vi "Declare_Sync_Client.vi"   [LabVIEW 2020]
uses:
  ADAM Client/Sub VIs/ADAM Controls/Channel_State.ctl
  ADAM Client/Sub VIs/ADAM Controls/Calib_type_ADAM.ctl
  ADAM Client/Sub VIs/ADAM Controls/Module_type_ADAM.ctl
  ADAM Client/Sub VIs/ADAM Controls/Ch_description_ADAM.ctl
  ADAM Client/Sub VIs/ADAM Controls/Function_ADAM.ctl
  ADAM Client/Sub VIs/ADAM Controls/Address.ctl
  ADAM Client/Sub VIs/ADAM Controls/Update_scan_value.ctl
  Globals/Preference_global.vi
types:
  T1 = typedef "Channel_State.ctl" = enum16{"On", "Off", "Always On", "Always Off"}
  T2 = typedef "Ch_description_ADAM.ctl" = cluster{"Ch Name":string, "Type":T3, "Function":T4, "Ch State":T1, "Calibration type":T5, "A":dbl, "B":dbl, "C":dbl, "D":dbl, "Comments":string, "Address":T6, "String":string, "Duty":u16}
  T3 = typedef "Module_type_ADAM.ctl" = string
  T4 = typedef "Function_ADAM.ctl" = enum16{"Analogue Input", "Digital Input", "Event counter", "Event rate", "Analogue Output", "Digital Output", "Relay Output"}
  T5 = typedef "Calib_type_ADAM.ctl" = string
  T6 = typedef "Address.ctl" = cluster{"Main":i32, "Ch.":i32, "Sub":i32, "Port Name":string}
  T7 = typedef "Update_scan_value.ctl" = cluster{"Channel Name":string, "New Value":dbl}
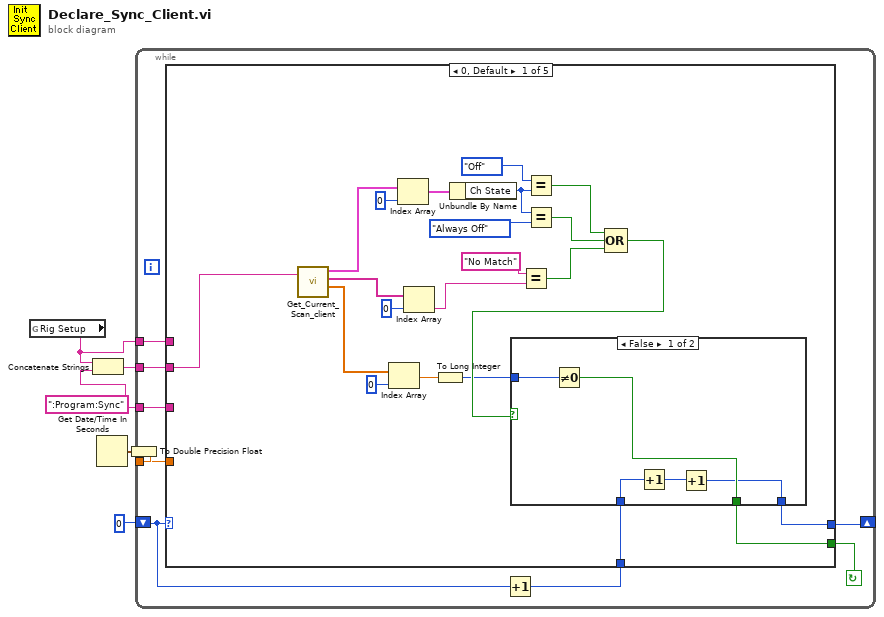
[diagram p0: block diagram]
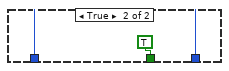
[diagram p2: hidden frame]
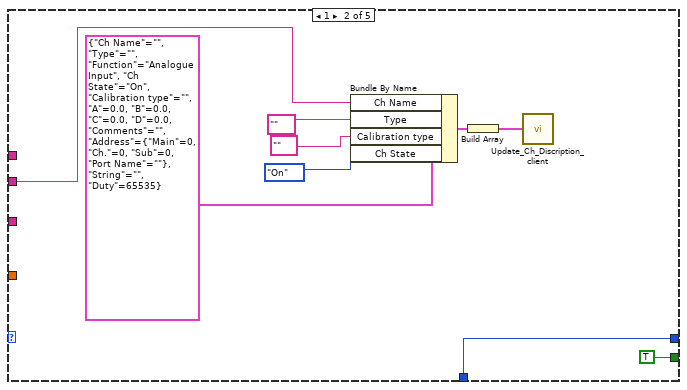
[diagram p3: hidden frame]
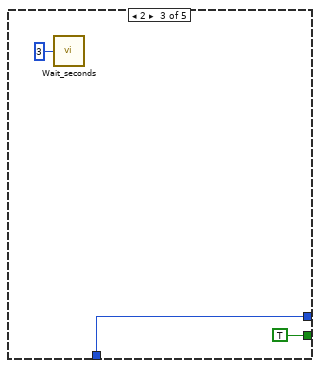
[diagram p4: hidden frame]
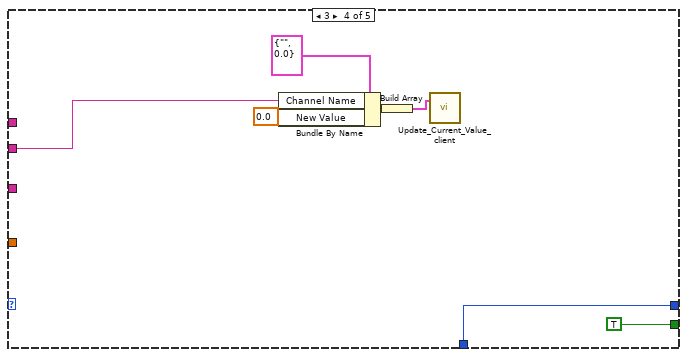
[diagram p5: hidden frame]
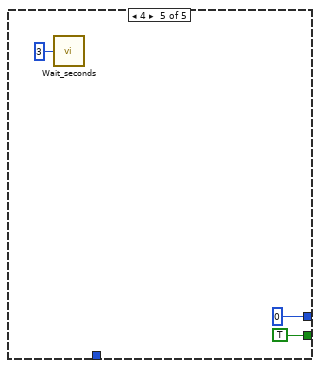
[diagram p6: hidden frame]
diagram:
  w5 = ":Program:Sync"
  n1 = global read "Preference_global.vi" "Rig Setup"() -> (w2:string)
  n2 = Concatenate Strings(w2, w5) -> (w4:string)
  n3 = Get Date/Time In Seconds() -> (seconds since 1Jan1904=w1:timestamp)
  n4 = To Double Precision Float(number=w1) -> (double precision float=w6:dbl)
  n5 = while {
    tunnel: w2 -> [w7]
    tunnel: w6 -> [w8]
    tunnel: w4 -> [w9]
    tunnel: w5 -> [w10]
    shift-left: 0 -> [w13]
    shift-right: [w12] -> _
    stop <- w14 continue-if-true
    n6 = Increment(x=w13) -> (x+1=w11:i32)
    n7 = case shown="0, Default" w13 {
      tunnel: [w16 TRUE TRUE TRUE TRUE] -> w14
      tunnel: [w21 w44 w55 w56 0] -> w12
      tunnel: w11 -> [w22 w44 w55 w56 _]
      tunnel: w10 -> [_ _ _ _ _]
      tunnel: w9 -> [w15 w45 _ w58 _]
      tunnel: w8 -> [_ _ _ _ _]
      tunnel: w7 -> [_ _ _ _ _]
      frame 0, Default {
        n8 = call "Get_Current_Scan_client.vi"("singleChannel"=w15) -> ("Ch Description Array"=w31:T2[], "String values"=w34:string[], "Numerical Values"=w19:dbl[])  [unwired: 1 in, 1 out]
        n9 = Index Array(array=w19, index=0 ("Index")) -> (element=w18:dbl)
        n10 = Index Array(array=w31, index=0 ("Index")) -> (element=w30:T2)
        n11 = Index Array(array=w34, index=0 ("Index")) -> (element=w33:string)
        n12 = To Long Integer(number=w18) -> (32bit integer=w17:i32)
        n13 = Unbundle By Name(w30) -> ("Ch State"=w28:T1)
        n14 = Equal?(x="No Match", y=w33) -> (x = y?=w24:bool)
        n15 = Equal?(x=Channel_State."Off" ("Ch State"), y=w28) -> (x = y?=w26:bool)
        n16 = Equal?(x=w28, y=Channel_State."Always Off" ("Ch State")) -> (x = y?=w25:bool)
        n17 = Compound Arithmetic op=OR(w26, w25, w24) -> (w23:bool)
        n18 = case shown="False" w23 {
          tunnel: w22 -> [w39 w43]
          tunnel: [w37 w43] -> w21
          tunnel: w17 -> [w41 _]
          tunnel: [w40 TRUE] -> w16
          frame False {
            n19 = Not Equal To 0?(x=w41) -> (x != 0?=w40:bool)
            n20 = Increment(x=w39) -> (x+1=w38:i32)
            n21 = Increment(x=w38) -> (x+1=w37:i32)
          }
          frame True {
          }
        }
      }
      frame 1 {
        n22 = Bundle By Name(cluster=T2 {"Ch Name"="", "Type"="", "Function"=enum."Analogue Input", "Ch State"=enum."On", "Calibration type"="", "A"=0.0, "B"=0.0, "C"=0.0, "D"=0.0, "Comments"="", "Address"={"Main"=0, "Ch."=0, "Sub"=0, "Port Name"=""}, "String"="", "Duty"=65535} ("Ch Discription"), "Ch Name"=w45, "Type"=T3 "", "Calibration type"=T5 "", "Ch State"=Channel_State."On") -> (w51:T2)
        n23 = Build Array(w51) -> (w52:T2[])
        n24 = call "Update_Ch_Discription_client.vi"("Channels to update In"=w52) -> ()  [unwired: 1 out]
      }
      frame 2 {
        n25 = call "Wait_seconds.vi"("Seconds to wait"=u32 3) -> ()
      }
      frame 3 {
        n26 = Bundle By Name(cluster=T7 {"Channel Name"="", "New Value"=0.0} ("Update Scan Value Cluster"), "Channel Name"=w58, "New Value"=0.0 ("Bundle Element")) -> (w61:T7)
        n27 = Build Array(w61) -> (w59:T7[])
        n28 = call "Update_Current_Value_client.vi"("Update array in"=w59) -> ()  [unwired: 1 in]
      }
      frame 4 {
        n29 = call "Wait_seconds.vi"("Seconds to wait"=u32 3) -> ()
      }
    }
  }
